vi "ArParser.vi"(1 "from\nXMLparser":string[][](array[string]), 2 "IndicatorClasses":string[](array[string]), 3 "IndicatorTypes":string[](array[string]), 4 "IndicatorNames":string[](array[string])) -> (0 "toCreator":T1(array[cluster]))   [LabVIEW 2010]
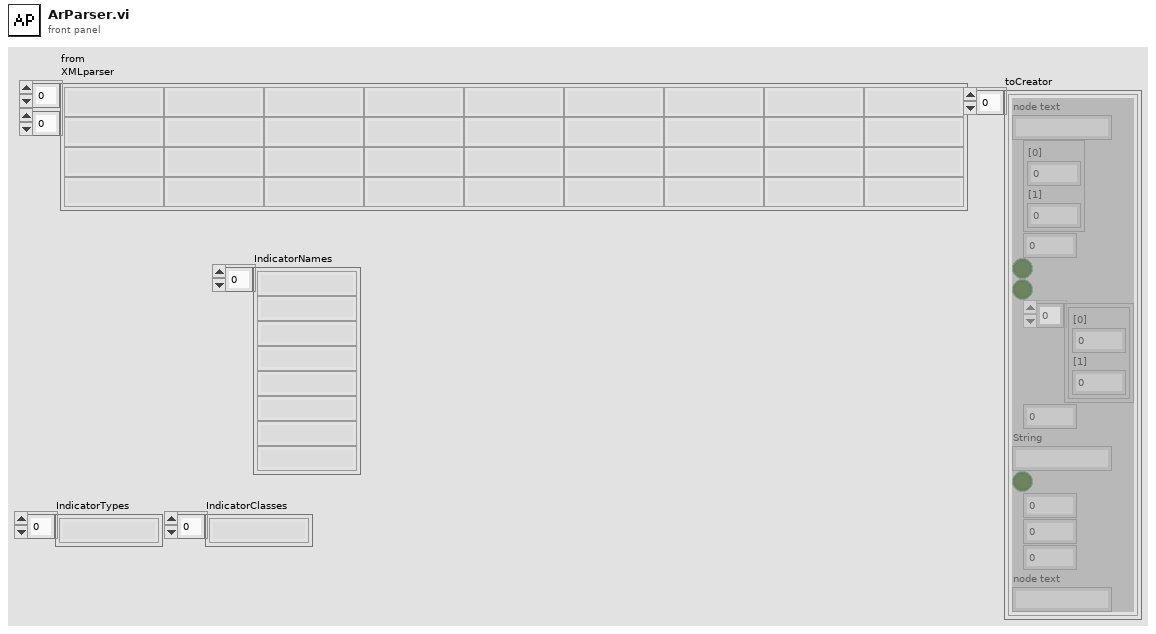
[diagram p1: front panel]
types:
  T1 = cluster{"node text":string, cluster{"[0]":i32, "[1]":i32}, i32, bool, bool, cluster{"[0]":u32, "[1]":u32}[], i32, "String":string, bool, i32, i32, i32, "node text":string}[]
  T2 = cluster{"node text":string, cluster{"[0]":i32, "[1]":i32}, "Numeric":i32, "Boolean":bool, "Boolean":bool, cluster{"[0]":u32, "[1]":u32}[], i32, "String":string, bool, "Numeric":i32, "Numeric":i32, "Numeric":i32, "node text":string}
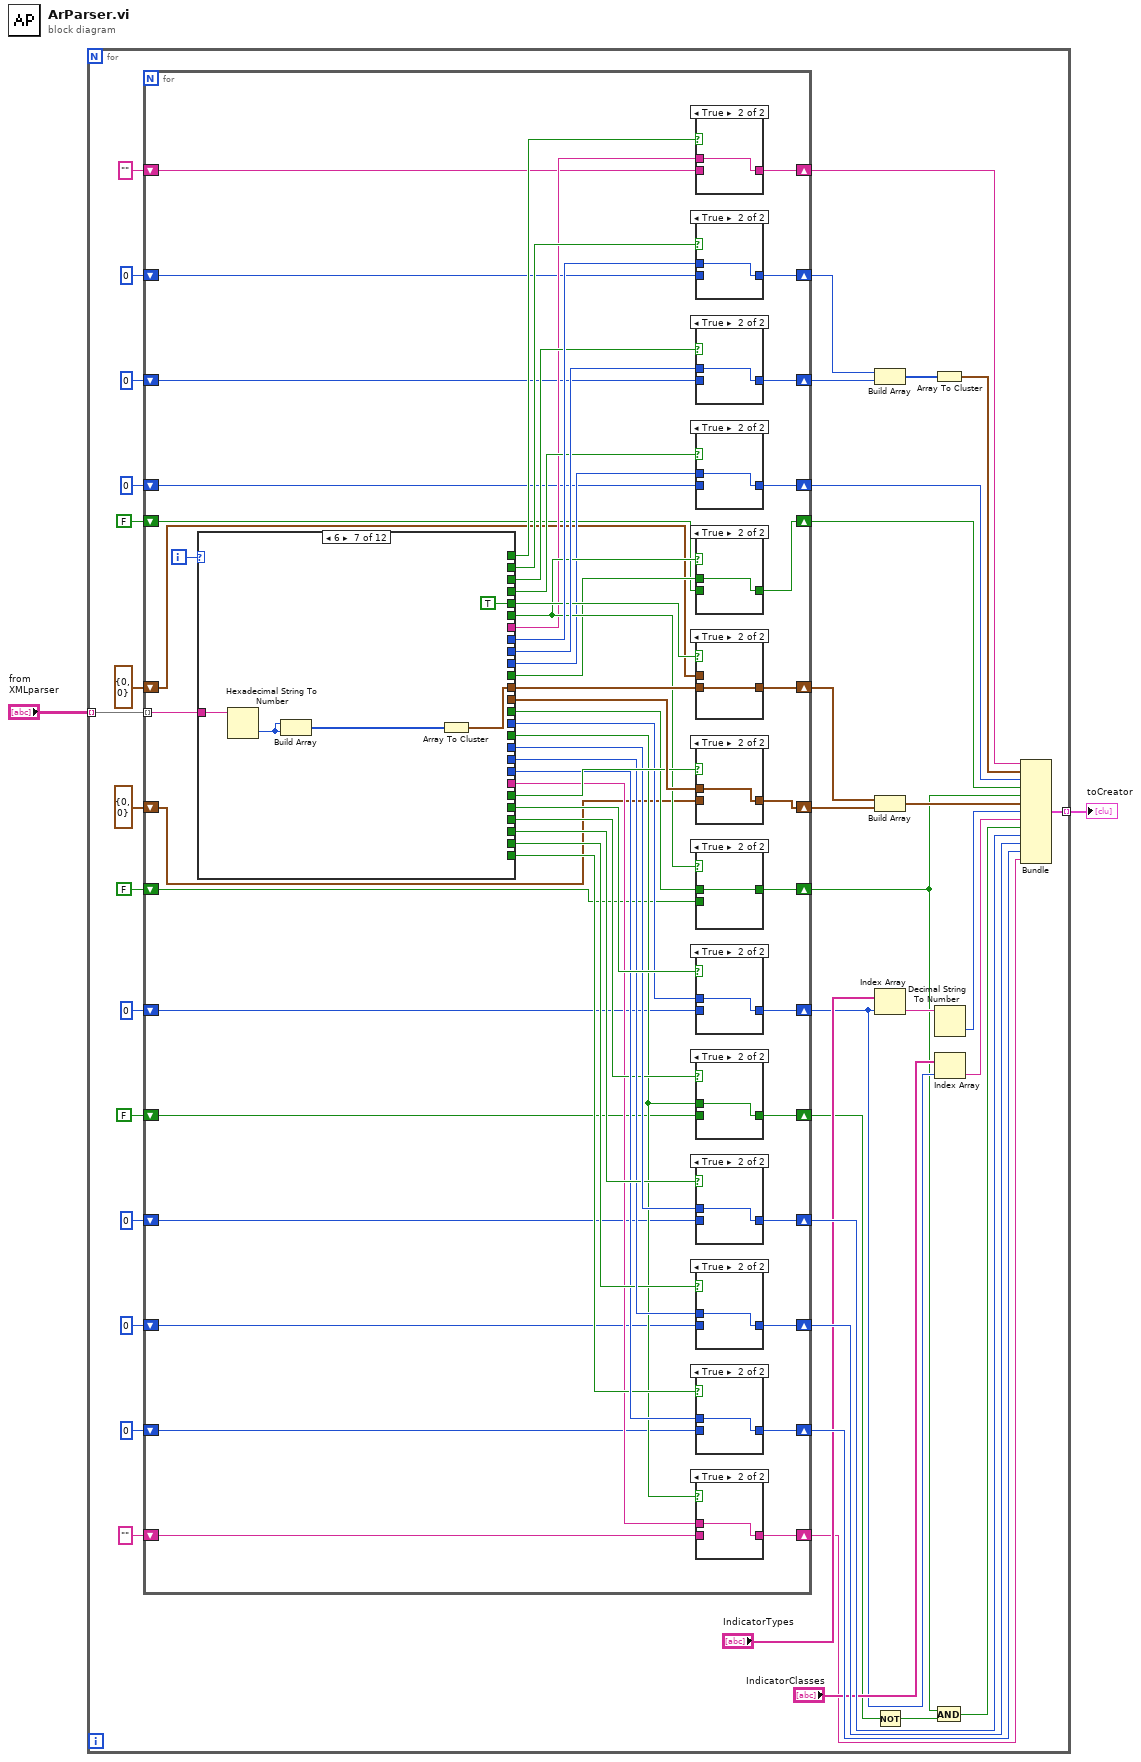
[diagram p0: block diagram]
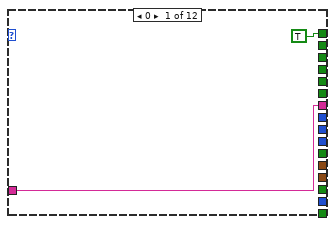
[diagram p16: hidden frame]
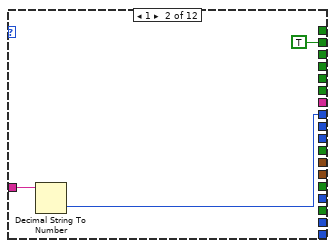
[diagram p17: hidden frame]
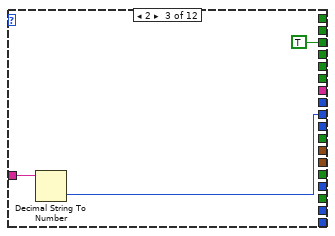
[diagram p18: hidden frame]
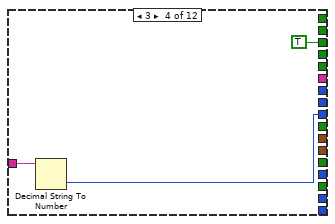
[diagram p19: hidden frame]
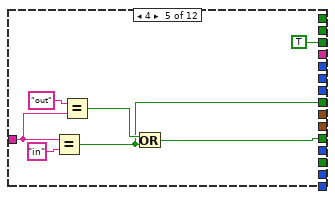
[diagram p20: hidden frame]
diagram:
  n1 = for {
    tunnel: "from\nXMLparser" -> [w42] mode=indexing
    tunnel: [w19] -> w1 mode=indexing
    n2 = for {
      tunnel: w42 -> [w98] mode=indexing
      shift-right: [w69] -> w18
      shift-left: "" ("node text") -> [w70]
      shift-right: [w67] -> w32
      shift-left: 0 ("Numeric") -> [w68]
      shift-right: [w65] -> w31
      shift-left: 0 ("Numeric") -> [w66]
      shift-right: [w63] -> w41
      shift-left: 0 ("Numeric") -> [w64]
      shift-right: [w61] -> w40
      shift-left: FALSE ("Boolean") -> [w62]
      shift-right: [w59] -> w35
      shift-left: cluster{"[0]":u32, "[1]":u32} {"[0]"=0, "[1]"=0} ("Cluster") -> [w60]
      shift-right: [w57] -> w34
      shift-left: cluster{"[0]":u32, "[1]":u32} {"[0]"=0, "[1]"=0} ("Cluster") -> [w58]
      shift-right: [w55] -> w21
      shift-left: FALSE ("Boolean") -> [w56]
      shift-right: [w53] -> w26
      shift-left: 0 ("index of element") -> [w54]
      shift-right: [w51] -> w39
      shift-left: 0 ("Numeric") -> [w52]
      shift-right: [w49] -> w38
      shift-left: 0 ("Numeric") -> [w50]
      shift-right: [w47] -> w37
      shift-left: 0 ("Numeric") -> [w48]
      shift-right: [w45] -> w23
      shift-left: FALSE ("Boolean") -> [w46]
      shift-right: [w43] -> w17
      shift-left: "" ("node text") -> [w44]
      i -> [w93]
      n3 = case shown="6" w93 {
        tunnel: w98 -> [w127 w131 w134 w137 w139 w149 w154 w158 w164 w167 w170 _]
        tunnel: [w127 _ _ _ _ _ _ _ _ _ _ _] -> w79
        tunnel: [_ w130 _ _ _ _ _ _ _ _ _ _] -> w97
        tunnel: [_ _ w133 _ _ _ _ _ _ _ _ _] -> w96
        tunnel: [_ _ _ w136 _ _ _ _ _ _ _ _] -> w85
        tunnel: [_ _ _ _ w138 _ _ _ _ _ _ _] -> w86
        tunnel: [_ _ _ _ _ w146 _ _ _ _ _ _] -> w95
        tunnel: [_ _ _ _ _ _ w151 _ _ _ _ _] -> w94
        tunnel: [TRUE _ _ _ _ _ _ _ _ _ _ _] -> w92
        tunnel: [_ _ _ _ TRUE _ _ _ _ _ _ _] -> w87
        tunnel: [_ _ _ _ _ TRUE _ _ _ _ _ _] -> w91
        tunnel: [_ _ _ _ _ _ TRUE _ _ _ _ _] -> w90
        tunnel: [_ TRUE _ _ _ _ _ _ _ _ _ _] -> w89
        tunnel: [_ _ TRUE _ _ _ _ _ _ _ _ _] -> w88
        tunnel: [_ _ _ TRUE _ _ _ _ _ _ _ _] -> w84
        tunnel: [_ _ _ _ w143 _ _ _ _ _ _ _] -> w78
        tunnel: [_ _ _ _ _ _ _ w160 _ _ _ _] -> w82
        tunnel: [_ _ _ _ _ _ _ w159 _ _ _ _] -> w83
        tunnel: [_ _ _ _ _ _ _ _ w163 _ _ _] -> w81
        tunnel: [_ _ _ _ _ _ _ _ TRUE _ _ _] -> w80
        tunnel: [_ _ _ _ _ _ _ _ _ w166 _ _] -> w77
        tunnel: [_ _ _ _ _ _ _ _ _ TRUE _ _] -> w76
        tunnel: [_ _ _ _ _ _ _ _ _ _ w169 _] -> w75
        tunnel: [_ _ _ _ _ _ _ _ _ _ TRUE _] -> w74
        tunnel: [_ _ _ _ _ _ _ w155 _ _ _ _] -> w71
        tunnel: [_ _ _ _ _ _ _ w159 _ _ _ _] -> w73
        tunnel: [_ _ _ _ _ _ _ w158 _ _ _ _] -> w72
        frame 0 {
        }
        frame 1 {
          n4 = Decimal String To Number(string=w131) -> (number=w130:i32)  [unwired: 2 in, 1 out]
        }
        frame 2 {
          n5 = Decimal String To Number(string=w134) -> (number=w133:i32)  [unwired: 2 in, 1 out]
        }
        frame 3 {
          n6 = Decimal String To Number(string=w137) -> (number=w136:i32)  [unwired: 2 in, 1 out]
        }
        frame 4 {
          n7 = Equal?(x=w139, y="in") -> (x = y?=w138:bool)
          n8 = Equal?(x="out", y=w139) -> (x = y?=w140:bool)
          n9 = Or(x=w140, y=w138) -> (x .or. y?=w143:bool)
        }
        frame 5 {
          n10 = Hexadecimal String To Number(string=w149) -> (number=w145:u32)  [unwired: 2 in, 1 out]
          n11 = Build Array(w145, w145) -> (w147:u32[])
          n12 = Array To Cluster(array=w147) -> (cluster=w146:cluster{"[0]":u32, "[1]":u32})
        }
        frame 6 {
          n13 = Hexadecimal String To Number(string=w154) -> (number=w150:u32)  [unwired: 2 in, 1 out]
          n14 = Build Array(w150, w150) -> (w152:u32[])
          n15 = Array To Cluster(array=w152) -> (cluster=w151:cluster{"[0]":u32, "[1]":u32})
        }
        frame 7 {
          w159 = TRUE
          n16 = Search 1D Array(1D array="IndicatorNames", element=w158) -> (index of element=w157:i32)  [unwired: 1 in]
          n17 = Increment(x=w157) -> (x+1=w156:i32)
          n18 = Less Than 0?(x=w157) -> (x < 0?=w155:bool)
          n19 = Select(t=w156, s=w155, f=w157) -> (s? t:f=w160:i32)
        }
        frame 8 {
          n20 = Decimal String To Number(string=w164) -> (number=w163:i32)  [unwired: 2 in, 1 out]
        }
        frame 9 {
          n21 = Decimal String To Number(string=w167) -> (number=w166:i32)  [unwired: 2 in, 1 out]
        }
        frame 10 {
          n22 = Decimal String To Number(string=w170) -> (number=w169:i32)  [unwired: 2 in, 1 out]
        }
        frame -1, Default {
        }
      }
      n23 = case shown="True" w92 {
        tunnel: w70 -> [w125 _]
        tunnel: w79 -> [_ w126]
        tunnel: [w125 w126] -> w69
        frame False {
        }
        frame True {
        }
      }
      n24 = case shown="True" w89 {
        tunnel: w68 -> [w123 _]
        tunnel: w97 -> [_ w124]
        tunnel: [w123 w124] -> w67
        frame False {
        }
        frame True {
        }
      }
      n25 = case shown="True" w88 {
        tunnel: w66 -> [w121 _]
        tunnel: w96 -> [_ w122]
        tunnel: [w121 w122] -> w65
        frame False {
        }
        frame True {
        }
      }
      n26 = case shown="True" w84 {
        tunnel: w64 -> [w119 _]
        tunnel: w85 -> [_ w120]
        tunnel: [w119 w120] -> w63
        frame False {
        }
        frame True {
        }
      }
      n27 = case shown="True" w87 {
        tunnel: w62 -> [w117 _]
        tunnel: w86 -> [_ w118]
        tunnel: [w117 w118] -> w61
        frame False {
        }
        frame True {
        }
      }
      n28 = case shown="True" w90 {
        tunnel: w58 -> [w113 _]
        tunnel: w94 -> [_ w114]
        tunnel: [w113 w114] -> w57
        frame False {
        }
        frame True {
        }
      }
      n29 = case shown="True" w91 {
        tunnel: w60 -> [w115 _]
        tunnel: w95 -> [_ w116]
        tunnel: [w115 w116] -> w59
        frame False {
        }
        frame True {
        }
      }
      n30 = case shown="True" w87 {
        tunnel: w56 -> [w111 _]
        tunnel: w78 -> [_ w112]
        tunnel: [w111 w112] -> w55
        frame False {
        }
        frame True {
        }
      }
      n31 = case shown="True" w83 {
        tunnel: w54 -> [w109 _]
        tunnel: w82 -> [_ w110]
        tunnel: [w109 w110] -> w53
        frame False {
        }
        frame True {
        }
      }
      n32 = case shown="True" w73 {
        tunnel: w46 -> [w101 _]
        tunnel: w71 -> [_ w102]
        tunnel: [w101 w102] -> w45
        frame False {
        }
        frame True {
        }
      }
      n33 = case shown="True" w80 {
        tunnel: w52 -> [w107 _]
        tunnel: w81 -> [_ w108]
        tunnel: [w107 w108] -> w51
        frame False {
        }
        frame True {
        }
      }
      n34 = case shown="True" w76 {
        tunnel: w50 -> [w105 _]
        tunnel: w77 -> [_ w106]
        tunnel: [w105 w106] -> w49
        frame False {
        }
        frame True {
        }
      }
      n35 = case shown="True" w74 {
        tunnel: w48 -> [w103 _]
        tunnel: w75 -> [_ w104]
        tunnel: [w103 w104] -> w47
        frame False {
        }
        frame True {
        }
      }
      n36 = case shown="True" w71 {
        tunnel: w44 -> [w99 _]
        tunnel: w72 -> [_ w100]
        tunnel: [w99 w100] -> w43
        frame False {
        }
        frame True {
        }
      }
    }
    n37 = Build Array(w32, w31) -> (w33:i32[])
    n38 = Build Array(w34, w35) -> (w36:cluster{"[0]":u32, "[1]":u32}[])
    n39 = Index Array(array="IndicatorTypes", index=w26) -> (element=w27:string)
    n40 = Not(x=w23) -> (.not. x?=w22:bool)
    n41 = Array To Cluster(array=w33) -> (cluster=w30:cluster{"[0]":i32, "[1]":i32})
    n42 = And(x=w21, y=w22) -> (x .and. y?=w20:bool)
    n43 = Decimal String To Number(string=w27) -> (number=w25:i32)  [unwired: 2 in, 1 out]
    n44 = Index Array(array="IndicatorClasses", index=w26) -> (element=w24:string)
    n45 = Bundle("node text"=w18, w30, "Numeric"=w41, "Boolean"=w40, "Boolean"=w21, w36, w25, "String"=w24, w20, "Numeric"=w39, "Numeric"=w38, "Numeric"=w37, "node text"=w17) -> (w19:T2)  [unwired: 1 in]
  }
  "toCreator" <- w1
